vi "Check Button.vi"(8 "error in (no error)":errorcluster, 9 "Message Values":string[](array[string]), 10 "队列":T1, 11 "Table":refnum<vi>) -> (0 "error out":errorcluster)   [LabVIEW 2017]
uses:
  Depends/AMC/subVIs/TypeDefs/amc_Message Queue.ctl
  Depends/AMC/subVIs/TypeDefs/amc_Message.ctl
  Depends/Tools/Keyed Array/Tools_KeyedArray KeyedArray.ctl
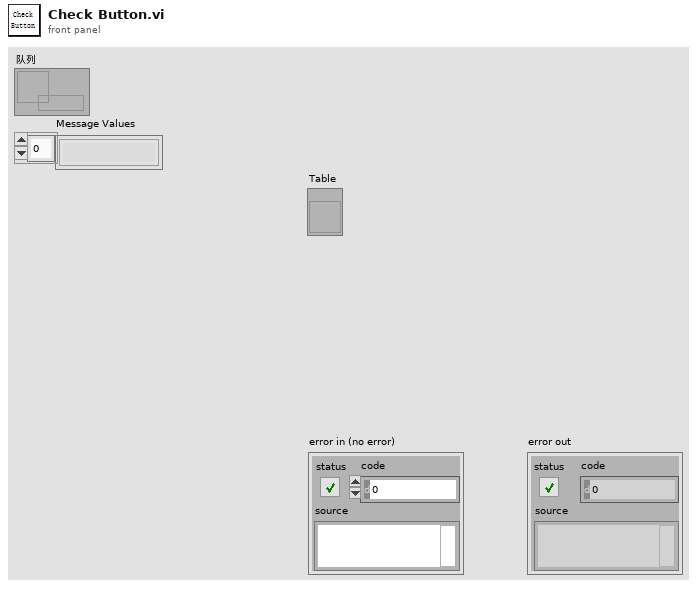
[diagram p1: front panel]
types:
  T1 = typedef "amc_Message Queue.ctl" = refnum<queue>
  T2 = typedef "SW Config.ctl" = cluster{"Station Name":string, "Station Code":string, "ES no.":string, "Station ID":string, "Certificate":path, "Fail-Stop":bool, "FFTesterPath":path, "Enable_User":bool, "T Number":string}
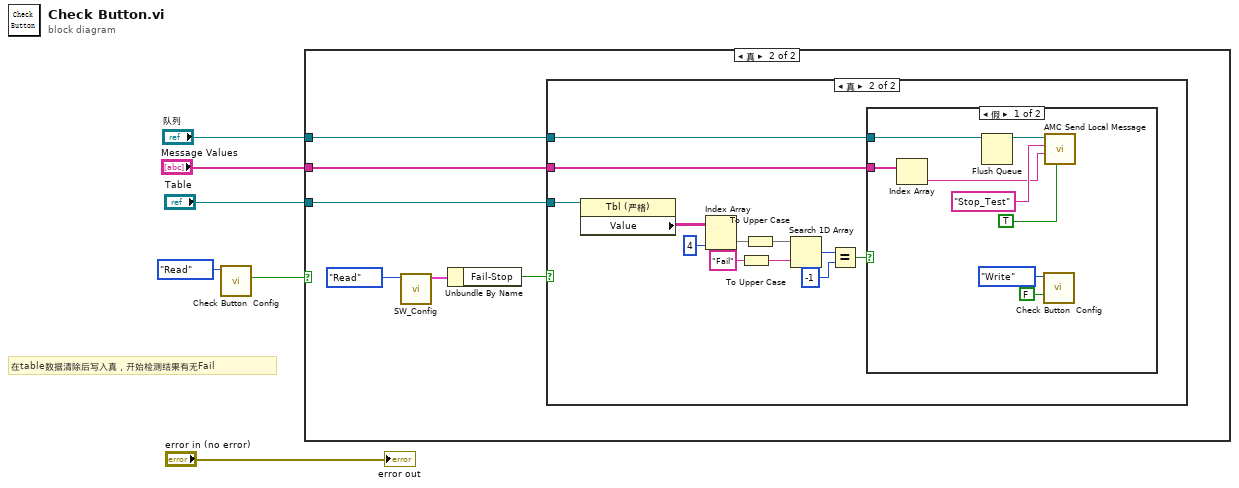
[diagram p0: block diagram]
diagram:
  # "在table数据清除后写入真，开始检测结果有无Fail"
  n1 = call "Check Button  Config.vi"("Step"=enum16{"Initial", "Write", "Read"}."Read") -> ("布尔 2"=w4:bool)  [unwired: 9 in, 1 out]
  n2 = case shown="真" w4 {
    tunnel: "Table" -> [_ w11]
    tunnel: "队列" -> [_ w10]
    tunnel: "Message Values" -> [_ w9]
    frame False {
    }
    frame True {
      n3 = call "SW_Config.vi"("Step"=enum16{"Initial", "Write", "Read"}."Read") -> ("SW Config out"=w7:T2)  [unwired: 9 in, 1 out]
      n4 = Unbundle By Name(w7) -> ("Fail-Stop"=w12:bool)
      n5 = case shown="真" w12 {
        tunnel: w11 -> [_ w24]
        tunnel: w10 -> [_ w16]
        tunnel: w9 -> [_ w15]
        frame False {
        }
        frame True {
          n6 = property class="Tbl (严格)"(reference=w24) -> ("Value"=w23:string[][])  [unwired: 1 in, 2 out]
          n7 = Index Array(array=w23, index (col)=4 ("禁用的索引 (列)")) -> (element=w21:string[])  [unwired: 1 in]
          n8 = To Upper Case(1:"Fail" ("元素")) -> (0:w13:string)
          n9 = To Upper Case(1:w21) -> (0:w14:string[])
          n10 = Search 1D Array(1D array=w14, element=w13) -> (index of element=w19:i32)  [unwired: 1 in]
          n11 = Equal?(x=w19, y=-1) -> (x = y?=w17:bool)
          n12 = case shown="假" w17 {
            tunnel: w16 -> [w29 _]
            tunnel: w15 -> [w26 _]
            frame False {
              n13 = Index Array(array=w26) -> (element=w25:string)  [unwired: 1 in]
              n14 = Flush Queue(queue=w29) -> (queue out=w30:T1)  [unwired: 1 in, 2 out]
              n15 = call "Check Button  Config.vi"("布尔"=FALSE, "Step"=enum16{"Initial", "Write", "Read"}."Write") -> ()  [unwired: 8 in, 2 out]
              n16 = call "AMC Send Local Message.vi"("Priority Message (F)"=TRUE, "Message Value"=w25, "Message Name"="Stop_Test", "Message Queue in"=w30) -> ()  [unwired: 6 in, 2 out]
            }
            frame True {
            }
          }
        }
      }
    }
  }
  "error out" <- "error in (no error)"
